vi "Where Do change.vi"(7 "Device Name":string, 10 "New Value":bool[][](array[boolean])=[[FALSE, FALSE, FALSE, FALSE, FALSE, FALSE, FALSE, FALSE], [FALSE, FALSE, FALSE, FALSE, FALSE, FALSE, FALSE, FALSE], [FALSE, FALSE, FALSE, FALSE, FALSE, FALSE, FALSE, FALSE], [FALSE, FALSE, FALSE, FALSE, FALSE, FALSE, FALSE, FALSE]], 11 "Old Value":bool[][](array[boolean])=[[FALSE, FALSE, FALSE, FALSE, FALSE, FALSE, FALSE, FALSE], [FALSE, FALSE, FALSE, FALSE, FALSE, FALSE, FALSE, FALSE], [FALSE, FALSE, FALSE, FALSE, FALSE, FALSE, FALSE, FALSE], [FALSE, FALSE, FALSE, FALSE, FALSE, FALSE, FALSE, FALSE]]) -> (3 "Out_prar":cluster{"Channel":string, "New_V":bool})   [LabVIEW 2017]
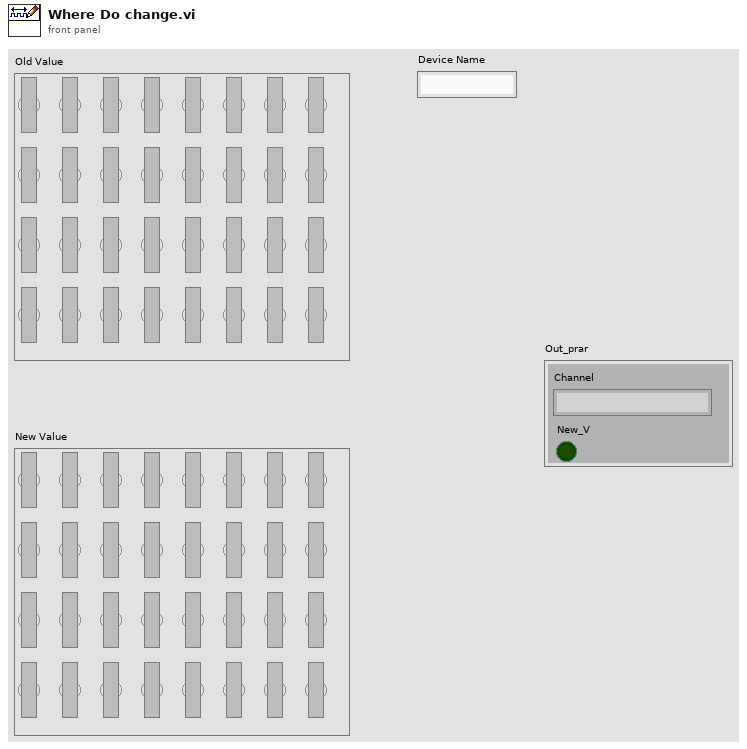
[diagram p1: front panel]
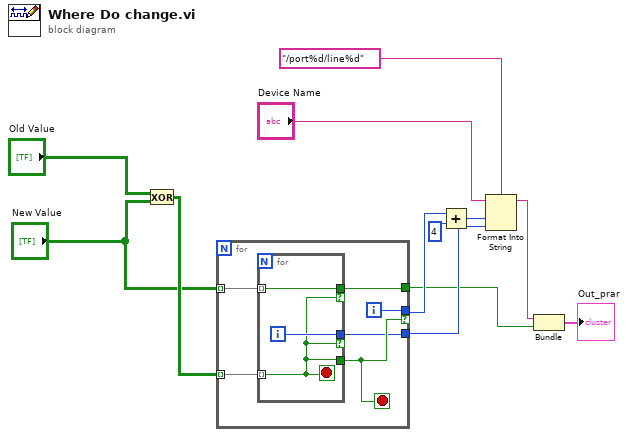
[diagram p0: block diagram]
diagram:
  n1 = Exclusive Or(1:"New Value", 2:"Old Value") -> (0:w11:bool[][])
  n2 = for {
    tunnel: w11 -> [w18] mode=indexing
    tunnel: [w17] -> w7 if=w16
    tunnel: "New Value" -> [w15] mode=indexing
    tunnel: [w14] -> w3
    tunnel: [w13] -> w6
    i -> [w17]
    stop <- w16 stop-if-true
    n3 = for {
      tunnel: w18 -> [w19] mode=indexing
      tunnel: [w21] -> w13 if=w19
      tunnel: [w19] -> w16
      tunnel: w15 -> [w20] mode=indexing
      tunnel: [w20] -> w14 if=w19
      i -> [w21]
      stop <- w19 stop-if-true
    }
  }
  n4 = Add(x=w7, y=4) -> (x+y=w2:i32)
  n5 = Format Into String(format string="/port%d/line%d", initial string="Device Name", w2, w6) -> (resulting string=w4:string)  [unwired: 1 in, 1 out]
  n6 = Bundle(w4, "Boolean"=w3) -> (→"Out_prar":cluster{string, "Boolean":bool})  [unwired: 1 in]
